vi "Client Viewer.vi"() -> ()   [LabVIEW 2009]
uses:
  UDP Lib/UDP Network Location.ctl
  <vilib>/Platform/TimedLoop/XDataNode/XDataNode.xnode
  <vilib>/Platform/TimedLoop/XDataNode/loadlvalarms.vi
  <vilib>/Platform/TimedLoop/XDataNode/timing_clust.ctl
  <vilib>/Platform/TimedLoop/XDataNode/nitl_modes.ctl
  <vilib>/Platform/TimedLoop/XDataNode/wakeup.ctl
  <vilib>/Platform/TimedLoop/XDataNode/XDNodeRunTimeDep.lvlib
panel:
  out "Keepalive":bool
  out "Timeout":bool
  in  "Destination Location":T1={"IP Address"="192.168.1.2", "Port"=50001}
  in  "Toggle":bool
  out "HB":bool
  out "Network Location":T1={"IP Address"="192.168.1.2", "Port"=50000}
  out "Count out":i32
  in  "stop":bool
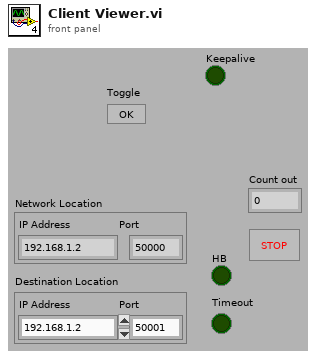
[diagram p1: front panel]
types:
  T1 = typedef "UDP Network Location.ctl" = cluster{"IP Address":string, "Port":u16}
  T2 = typedef "UDP Base.ctl" = cluster{"UDP Session":refnum<k16>, "UDP Socket Params":T3}
  T3 = typedef "UDP Socket Params.ctl" = cluster{"Local Port":u16, "Read Timeout":i32, "Write Timeout":i32}
  T4 = typedef "XDNodeRunTimeDep.lvlib/timing_clust.ctl" = cluster{"Expected End [f-1]":u64, "Actual End [f-1]":u64, "Finished Late? [f-1]":bool, "Expected End [i-1]":u64, "Actual End [i-1]":u64, "Finished Late? [i-1]":bool, "Expected Start [i]":u64, "Actual Start [i]":u64, "Expected Start [f]":u64, "Actual Start [f]":u64, "Source Name":string, "Structure Name":string, "Period":i64, "Deadline":i64, "Offset":i64, "Start":i64, "Priority":i32, "Timeout":i32, "Mode":T5, "Wakeup Reason":T6, "Error":errorcluster, "Source Type":string, "Secondary Source Type":string, "Global End Time":u64, "Global Start Time":u64, "Frame Duration":u64, "Iteration Duration":u64, "Assigned CPU":i32, "I/O Scan Engine Mode":u32}
  T5 = typedef "XDNodeRunTimeDep.lvlib/nitl_modes.ctl" = enum32{"No Change", "Process missed periods, maintain original phase", "Discard missed periods, maintain original phase", "Process missed periods, ignore original phase", "Discard missed periods, ignore original phase"}
  T6 = typedef "XDNodeRunTimeDep.lvlib/wakeup.ctl" = enum32{"Normal", "Aborted", "Asynchronous wakeup", "Timing source error", "Timed loop error", "Timeout"}
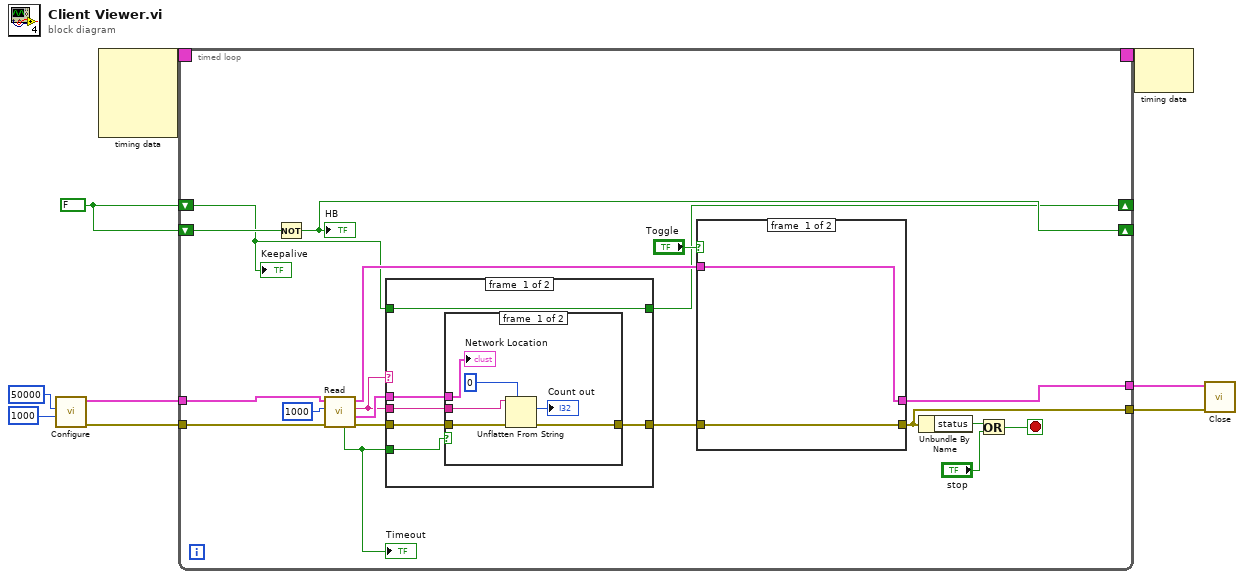
[diagram p0: block diagram]
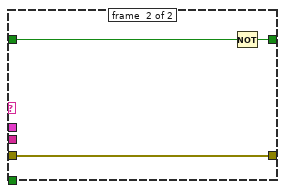
[diagram p3: hidden frame]
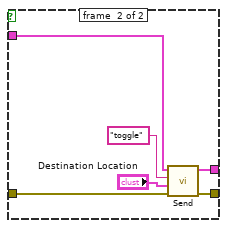
[diagram p4: hidden frame]
diagram:
  w1 = FALSE ("Timeout")
  n1 = call "Configure.vi"("Read Timeout"=1000, "Local Port"=u16 50000) -> ("error out"=w4:errorcluster, "UDP Base out"=w5:T2)  [unwired: 8 in]
  n2 = node-c288() -> (w9:T4)  [unwired: 4 in]
  n3 = timed-loop {
    timing: w9 -> [_]
    timing-out: [_] -> w8
    tunnel: [w15] -> w7
    tunnel: [w14] -> w6
    tunnel: w5 -> [w27]
    tunnel: w4 -> [w26]
    shift-right: [w22] -> _
    shift-left: w1 -> [w23]
    shift-right: [w11] -> _
    shift-left: w1 -> [w10]
    stop <- w21 stop-if-true
    n4 = Not(x=w23) -> (.not. x?=w22:bool)
    "HB" <- w22
    n5 = call "Read.vi"("error in (no error)"=w26, "max size (548)"=1000, "UDP Base in"=w27) -> ("error out"=w25:errorcluster, "Network Location"=w28:T1, "Receive Data"=w12:string, "UDP Base out"=w16:T2, "Timeout"=w24:bool)  [unwired: 3 in, 1 out]
    "Timeout" <- w24
    n6 = case shown="Default" w12 {
      tunnel: w12 -> [w34 _]
      tunnel: w28 -> [w33 _]
      tunnel: w25 -> [w32 w44]
      tunnel: w24 -> [w31 _]
      tunnel: [w30 w44] -> w13
      tunnel: w10 -> [w29 w43]
      tunnel: [w29 w42] -> w11
      frame #0 {
        n7 = case shown="False" w31 {
          tunnel: w34 -> [w40 _]
          tunnel: w33 -> [w39 _]
          tunnel: w32 -> [w36 w41]
          tunnel: [w35 w41] -> w30
          frame #0 {
            n8 = Unflatten From String(type=0 ("Count out"), binary string=w40, error in (no error)=w36) -> (value=→"Count out":i32, error out=w35:errorcluster)  [unwired: 2 in, 1 out]
            "Network Location" <- w39
          }
          frame #1 {
          }
        }
      }
      frame #1 {
        n9 = Not(x=w43) -> (.not. x?=w42:bool)
      }
    }
    n10 = case shown="True" "Toggle" {
      tunnel: w13 -> [w46 w52]
      tunnel: w16 -> [w45 w51]
      tunnel: [w45 w50] -> w15
      tunnel: [w46 w47] -> w14
      frame #0 {
      }
      frame #1 {
        n11 = call "Send.vi"("error in (no error)"=w52, "Destination Location"="Destination Location", "Send Data"="toggle", "UDP Base in"=w51) -> ("error out"=w47:errorcluster, "UDP Base out"=w50:T2)  [unwired: 5 in, 1 out]
      }
    }
    n12 = Unbundle By Name(w14) -> ("status"=w20:bool)
    n13 = Or(x=w20, y="stop") -> (x .or. y?=w21:bool)
    "Keepalive" <- w10
  }
  n14 = node-c288(w8) -> ()  [unwired: 1 out]
  n15 = call "Close.vi"("error in (no error)"=w6, "Cluster of class private data"=w7) -> ()  [unwired: 9 in, 1 out]
